vi "Merge EQ parcials.vi"(8 "EQ DATA + REPORT (partial EQ)":u32[](array[numeric]) format="%.0x", 9 "Last Pixel":u32 max=99, 10 "First Pixel":u32 max=99, 11 "all EQ DATA + REPORT in":u32[](array[numeric]) format="%.0x") -> (2 "all EQ DATA + REPORT out":u32[](array[numeric]) format="%.0x")   [LabVIEW 2015, in "VIPM2.lvlib"]
doc: "In VIPauto, merge the 7 partial equalizations in only one \"all EQ DATA + REPORT (1 Layer)\".\nIn each execution of this VI, a partial equalization is added into the merged output.\nNomes funciona en el cas d'una Layer."
uses:
  VIPM2.lvlib
panel:
  # "Merge partial equalizations"
  # "In VIPauto, merge the 7 partial equalizations in only one \"all EQ DATA + REPORT (1 Layer)\".\nIn each execution of this VI, a partial equalization is added into the merged output.\nNomes funciona en el cas d'una Layer."
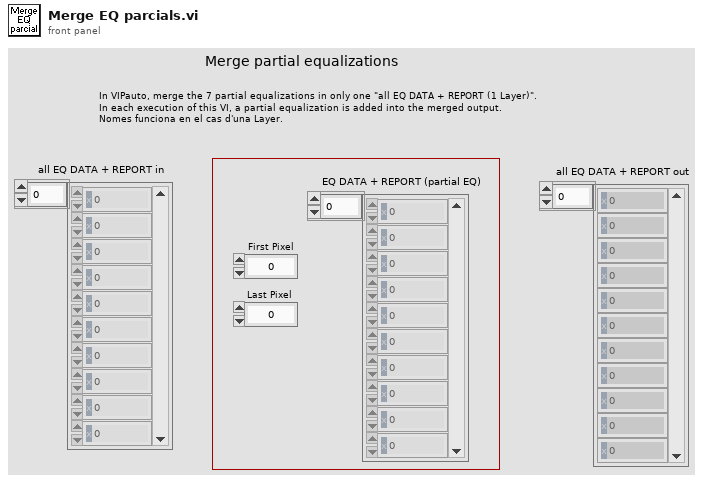
[diagram p1: front panel]
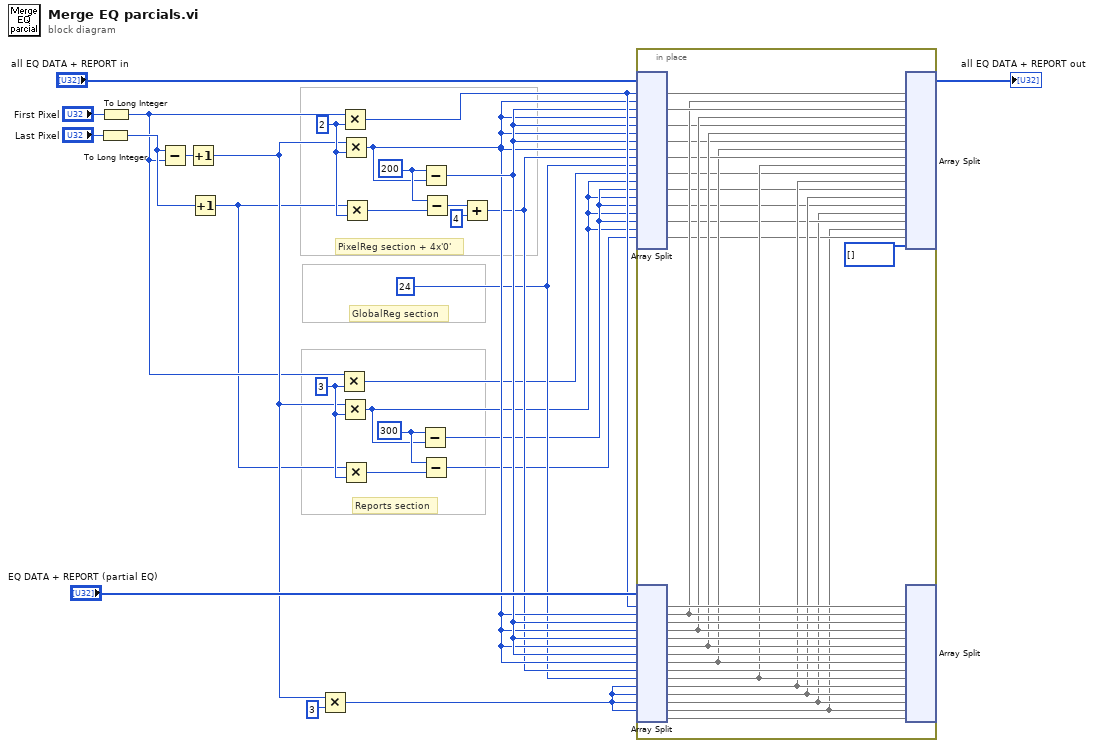
[diagram p0: block diagram]
diagram:
  w8 = 300 ("x")
  w9 = 3 ("y")
  w13 = 24
  w23 = 200 ("x")
  w22 = 2 ("y")
  # "Reports section"
  # "GlobalReg section"
  # "PixelReg section + 4x'0'"
  n1 = To Long Integer(number="Last Pixel") -> (32bit integer=w20:i32)
  n2 = To Long Integer(number="First Pixel") -> (32bit integer=w6:i32)
  n3 = Subtract(x=w20, y=w6) -> (x-y=w26:i32)
  n4 = Increment(x=w26) -> (x+1=w7:i32)
  n5 = Increment(x=w20) -> (x+1=w5:i32)
  n6 = Multiply(x=w7, y=3) -> (x*y=w11:i32)
  n7 = Multiply(x=w6, y=w9) -> (x*y=w4:i32)
  n8 = Multiply(x=w6, y=w22) -> (x*y=w17:i32)
  n9 = Multiply(x=w7, y=w9) -> (x*y=w2:i32)
  n10 = Multiply(x=w7, y=w22) -> (x*y=w15:i32)
  n11 = Multiply(x=w5, y=w9) -> (x*y=w10:i32)
  n12 = Multiply(x=w5, y=w22) -> (x*y=w21:i32)
  n13 = Subtract(x=w8, y=w2) -> (x-y=w3:i32)
  n14 = Subtract(x=w23, y=w15) -> (x-y=w16:i32)
  n15 = Subtract(x=w8, y=w10) -> (x-y=w1:i32)
  n16 = Subtract(x=w23, y=w21) -> (x-y=w19:i32)
  n17 = Add(x=w19, y=4) -> (x+y=w14:i32)
  n18 = in-place "In Place Element Structure" {
    n19 = in-place-split #1("all EQ DATA + REPORT in", w17, w15, w16, w15, w16, w15, w16, w15, w14, w13, w4, w2, w3, w2, w3, w2, w3, w2, w1) -> (w55:u32[], w53:u32[], w49:u32[], w46:u32[], w44:u32[], w39:u32[], w37:u32[], w35:u32[], w34:u32[], w32:u32[])  [unwired: 10 out]
    n20 = in-place-split #2("EQ DATA + REPORT (partial EQ)", w17, w15, w16, w15, w16, w15, w16, w15, w14, w13, w11, w11, w11, w11) -> (w54:u32[], w52:u32[], w51:u32[], w50:u32[], w48:u32[], w47:u32[], w45:u32[], w43:u32[], w42:u32[], w41:u32[], w38:u32[], w36:u32[], w33:u32[], w30:u32[], w40:u32[])
    n21 = in-place-split #1(w55, w52, w53, w50, w49, w47, w46, w43, w44, w41, w39, w38, w37, w36, w35, w33, w34, w30, w32, u32[] [] ("subarray")) -> (→"all EQ DATA + REPORT out":u32[])  [unwired: 19 out]
    n22 = in-place-split #2(w54, w52, w51, w50, w48, w47, w45, w43, w42, w41, w38, w36, w33, w30, w40) -> ()  [unwired: 15 out]
  }
